vi "Motion-FindHome.vi"(8 "error in (no error)":errorcluster, 11 "Motion-ControlAll in":refnum<class "Motion-ControlAll.lvclass">) -> (0 "error out":errorcluster, 3 "Motion-ControlAll out":refnum<class "Motion-ControlAll.lvclass">)   [LabVIEW 2013, in "Motion-ControlAll.lvclass"]
uses:
  Motion-ControlAll.lvclass
  Motion-ControlAll.lvclass/Motion-ControlAll.ctl
  <vilib>/addons/_LabVIEW Style Book/Utilities/Style Book Utilities.lvlib
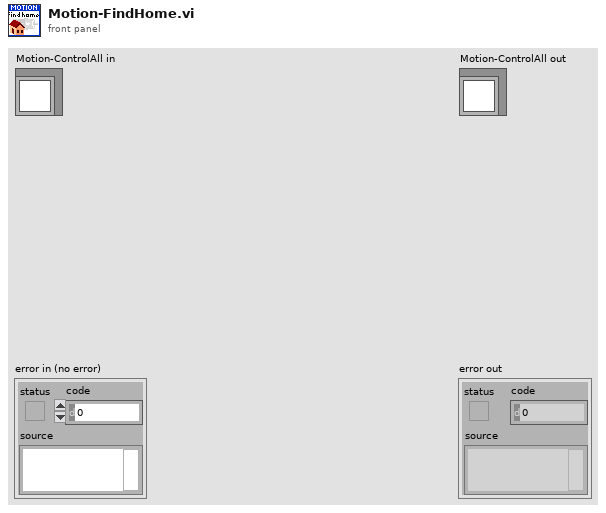
[diagram p1: front panel]
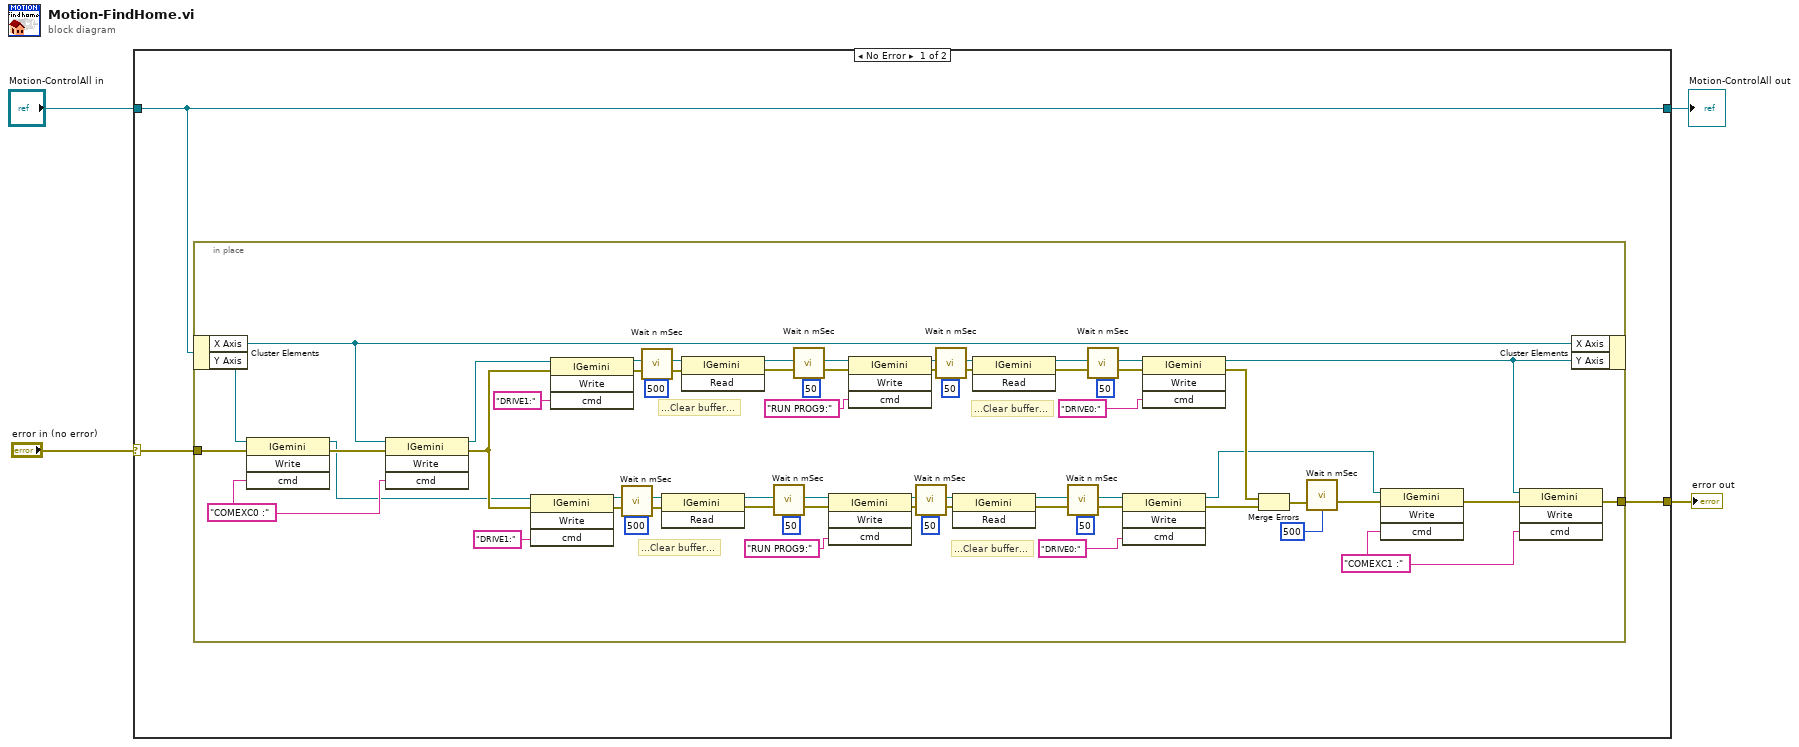
[diagram p0: block diagram]
diagram:
  n1 = case shown="No Error" "error in (no error)" {
    selector: "error in (no error)" -> [w6 w65]
    tunnel: [w5 w65] -> w3
    tunnel: [w7 w64] -> w1
    tunnel: "Motion-ControlAll in" -> [w7 w64]
    frame No Error {
      n2 = in-place {
        in-place-border: w6 -> [w20]
        in-place-border: [w8] -> w5
        w13 = "COMEXC1 :" ("cmd")
        w23 = "COMEXC0 :" ("cmd")
        # "...Clear buffer..."
        # "...Clear buffer..."
        # "...Clear buffer..."
        # "...Clear buffer..."
        n3 = in-place-cluster #1(w7) -> ("X Axis"=w10:refnum<k7>, "Y Axis"=w21:refnum<k7>)
        n4 = invoke class="IGemini" method="Write"(reference=w21, error in=w20, "cmd"=w23) -> (reference out=w17:refnum<k7>, error out=w22:errorcluster)  [unwired: 1 in, 2 out]
        n5 = invoke class="IGemini" method="Write"(reference=w10, error in=w22, "cmd"=w23) -> (reference out=w18:refnum<k7>, error out=w19:errorcluster)  [unwired: 1 in, 2 out]
        n6 = invoke class="IGemini" method="Write"(reference=w17, error in=w19, "cmd"="DRIVE1:" ("concatenated string")) -> (reference out=w26:refnum<k7>, error out=w27:errorcluster)  [unwired: 1 in, 2 out]
        n7 = invoke class="IGemini" method="Write"(reference=w18, error in=w19, "cmd"="DRIVE1:" ("concatenated string")) -> (reference out=w63:refnum<k7>, error out=w62:errorcluster)  [unwired: 1 in, 2 out]
        n8 = call <vilib>:"Wait n mSec.vi"("error in (no error)"=w27, "Milliseconds to Wait (500)"=u32 500) -> ("error out"=w28:errorcluster)  [unwired: 13 in]
        n9 = call <vilib>:"Wait n mSec.vi"("error in (no error)"=w62, "Milliseconds to Wait (500)"=u32 500) -> ("error out"=w61:errorcluster)  [unwired: 13 in]
        n10 = invoke class="IGemini" method="Read"(reference=w26, error in=w28) -> (reference out=w34:refnum<k7>, error out=w31:errorcluster)  [unwired: 1 in, 1 out]
        n11 = invoke class="IGemini" method="Read"(reference=w63, error in=w61) -> (reference out=w55:refnum<k7>, error out=w58:errorcluster)  [unwired: 1 in, 1 out]
        n12 = call <vilib>:"Wait n mSec.vi"("error in (no error)"=w31, "Milliseconds to Wait (500)"=u32 50) -> ("error out"=w33:errorcluster)  [unwired: 13 in]
        n13 = call <vilib>:"Wait n mSec.vi"("error in (no error)"=w58, "Milliseconds to Wait (500)"=u32 50) -> ("error out"=w56:errorcluster)  [unwired: 13 in]
        n14 = invoke class="IGemini" method="Write"(reference=w34, error in=w33, "cmd"="RUN PROG9:" ("concatenated string")) -> (reference out=w36:refnum<k7>, error out=w39:errorcluster)  [unwired: 1 in, 2 out]
        n15 = invoke class="IGemini" method="Write"(reference=w55, error in=w56, "cmd"="RUN PROG9:" ("concatenated string")) -> (reference out=w53:refnum<k7>, error out=w50:errorcluster)  [unwired: 1 in, 2 out]
        n16 = call <vilib>:"Wait n mSec.vi"("error in (no error)"=w39, "Milliseconds to Wait (500)"=u32 50) -> ("error out"=w37:errorcluster)  [unwired: 13 in]
        n17 = call <vilib>:"Wait n mSec.vi"("error in (no error)"=w50, "Milliseconds to Wait (500)"=u32 50) -> ("error out"=w52:errorcluster)  [unwired: 13 in]
        n18 = invoke class="IGemini" method="Read"(reference=w36, error in=w37) -> (reference out=w43:refnum<k7>, error out=w44:errorcluster)  [unwired: 1 in, 1 out]
        n19 = invoke class="IGemini" method="Read"(reference=w53, error in=w52) -> (reference out=w46:refnum<k7>, error out=w45:errorcluster)  [unwired: 1 in, 1 out]
        n20 = call <vilib>:"Wait n mSec.vi"("error in (no error)"=w44, "Milliseconds to Wait (500)"=u32 50) -> ("error out"=w41:errorcluster)  [unwired: 13 in]
        n21 = call <vilib>:"Wait n mSec.vi"("error in (no error)"=w45, "Milliseconds to Wait (500)"=u32 50) -> ("error out"=w48:errorcluster)  [unwired: 13 in]
        n22 = invoke class="IGemini" method="Write"(reference=w43, error in=w41, "cmd"="DRIVE0:" ("concatenated string")) -> (reference out=w11:refnum<k7>, error out=w24:errorcluster)  [unwired: 1 in, 2 out]
        n23 = invoke class="IGemini" method="Write"(reference=w46, error in=w48, "cmd"="DRIVE0:" ("concatenated string")) -> (reference out=w9:refnum<k7>, error out=w25:errorcluster)  [unwired: 1 in, 2 out]
        n24 = Merge Errors(w25, w24) -> (w16:errorcluster)
        n25 = call <vilib>:"Wait n mSec.vi"("error in (no error)"=w16, "Milliseconds to Wait (500)"=u32 500) -> ("error out"=w12:errorcluster)  [unwired: 13 in]
        n26 = invoke class="IGemini" method="Write"(reference=w11, error in=w12, "cmd"=w13) -> (error out=w14:errorcluster)  [unwired: 1 in, 3 out]
        n27 = invoke class="IGemini" method="Write"(reference=w9, error in=w14, "cmd"=w13) -> (error out=w8:errorcluster)  [unwired: 1 in, 3 out]
        n28 = in-place-cluster #1("X Axis"=w10, "Y Axis"=w9) -> ()  [unwired: 1 out]
      }
    }
    frame Error {
    }
  }
  "error out" <- w3
  "Motion-ControlAll out" <- w1
